vi "Limit Switch Check.vi"(11 "Input Cluster":T1) -> (3 "Output Cluster":T1)   [LabVIEW 2019]
uses:
  Implementation/Turrent Controller Typedef.ctl
  <vilib>/Rock Robotics/WPI/MotorControl/WPI_MotorControlDeviceRef.ctl
  <vilib>/Rock Robotics/WPI/MotorControl/WPI_MotorControlType.ctl
  <vilib>/Rock Robotics/SystemInterfaces/DIO/FPGA_DIOPWMChannel.ctl
  <vilib>/Rock Robotics/WPI/PWM/WPI_PWMDeadband.ctl
  <vilib>/Rock Robotics/SystemInterfaces/DIO/FPGA_DIOChannel.ctl
  <vilib>/Rock Robotics/SystemInterfaces/DutyCycle/FPGA_DutyCycleDevRef.ctl
  <vilib>/Rock Robotics/SystemInterfaces/DutyCycle/FPGA_DutyCycleIndex.ctl
  <vilib>/Rock Robotics/WPI/Counter/WPI_CounterDevRef.ctl
  <vilib>/Rock Robotics/SystemInterfaces/Counter/FPGA_CounterCtrSystemIndex.ctl
  <vilib>/Rock Robotics/WPI/ThirdParty/REV Robotics/SPARK MAX/Typedef/Spark MAX Control Type.ctl
  Support Code/Indicator LED Indexes.ctl
  Support Code/Indicator LED - Green.ctl
panel:
  out "Hard Limit Fwd":bool
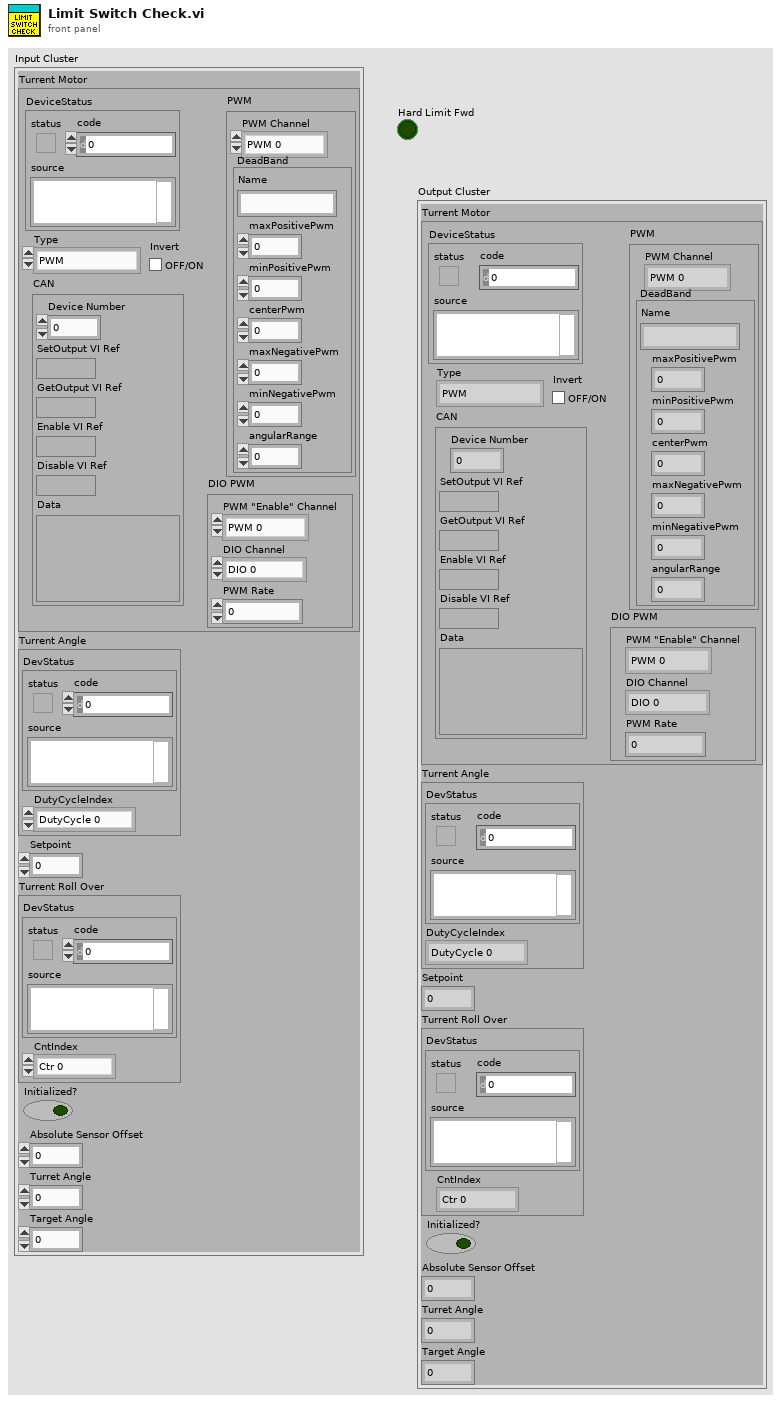
[diagram p1: front panel]
types:
  T1 = typedef "Turrent Controller Typedef.ctl" = cluster{"Turrent Motor":T2, "Turrent Angle":T7, "Setpoint":dbl, "Turrent Roll Over":T9, "Initialized?":bool, "Absolute Sensor Offset":dbl, "Turret Angle":dbl, "Target Angle":dbl}
  T2 = typedef "WPI_MotorControlDeviceRef.ctl" = cluster{"DeviceStatus":errorcluster, "Type":T3, "PWM":cluster{"PWM Channel":T4, "DeadBand":T5}, "CAN":cluster{"Device Number":u8, "SetOutput VI Ref":variant, "GetOutput VI Ref":variant, "Enable VI Ref":variant, "Disable VI Ref":variant, "Data":variant}, "Invert":bool, "DIO PWM":cluster{"PWM \"Enable\" Channel":T4, "DIOChannel":T6, "PWM Rate":dbl}}
  T3 = typedef "WPI_MotorControlType.ctl" = enum16{"PWM", "CAN", "DIO PWM"}
  T4 = typedef "FPGA_DIOPWMChannel.ctl" = enum8{"PWM 0", "PWM 1", "PWM 2", "PWM 3", "PWM 4", "PWM 5", "PWM 6", "PWM 7", "PWM 8", "PWM 9", "PWM MXP 0", "PWM MXP 1", "PWM MXP 2", "PWM MXP 3", "PWM MXP 4", "PWM MXP 5", "PWM MXP 6", "PWM MXP 7", "PWM MXP 8", "PWM MXP 9", "Invalid"}
  T5 = typedef "WPI_PWMDeadband.ctl" = cluster{"Name":string, "maxPositivePwm":i32, "minPositivePwm":i32, "centerPwm":i32, "maxNegativePwm":i32, "minNegativePwm":i32, "angularRange":u16}
  T6 = typedef "FPGA_DIOChannel.ctl" = enum8{"DIO 0", "DIO 1", "DIO 2", "DIO 3", "DIO 4", "DIO 5", "DIO 6", "DIO 7", "DIO 8", "DIO 9", "DIO MXP 0", "DIO MXP 1", "DIO MXP 2", "DIO MXP 3", "DIO MXP 4", "DIO MXP 5", "DIO MXP 6", "DIO MXP 7", "DIO MXP 8", "DIO MXP 9", "DIO MXP 10", "DIO MXP 11", "DIO MXP 12", "DIO MXP 13", "DIO MXP 14", "DIO MXP 15", "SPI Port CS1", "SPI Port CS2", "SPI Port CS3", "SPI Port MISO", "SPI Port MOSI", "Invalid"}
  T7 = typedef "FPGA_DutyCycleDevRef.ctl" = cluster{"DevStatus":errorcluster, "DutyCycleIndex":T8}
  T8 = typedef "FPGA_DutyCycleIndex.ctl" = enum8{"DutyCycle 0", "DutyCycle 1", "DutyCycle 2", "DutyCycle 3", "DutyCycle 4", "DutyCycle 5", "DutyCycle 6", "DutyCycle 7", "Invalid"}
  T9 = typedef "WPI_CounterDevRef.ctl" = cluster{"DevStatus":errorcluster, "CntIndex":T10}
  T10 = typedef "FPGA_CounterCtrSystemIndex.ctl" = enum8{"Ctr 0", "Ctr 1", "Ctr 2", "Ctr 3", "Ctr 4", "Ctr 5", "Ctr 6", "Ctr 7", "Invalid"}
  T11 = typedef "Spark MAX Control Type.ctl" = enum16{"Percent VBus", "Voltage", "Velocity", "Position", "Smart Motion", "Current", "Smart Velocity"}
  T12 = typedef "Indicator LED - Green.ctl" = u32
  T13 = typedef "Indicator LED Indexes.ctl" = enum16{"Code Started", "DS Connected", "Limelight", "Turret Calibrated", "Gyro Calibrated", "USB0 Connected", "USB1 Connected", "FMS Attached"}
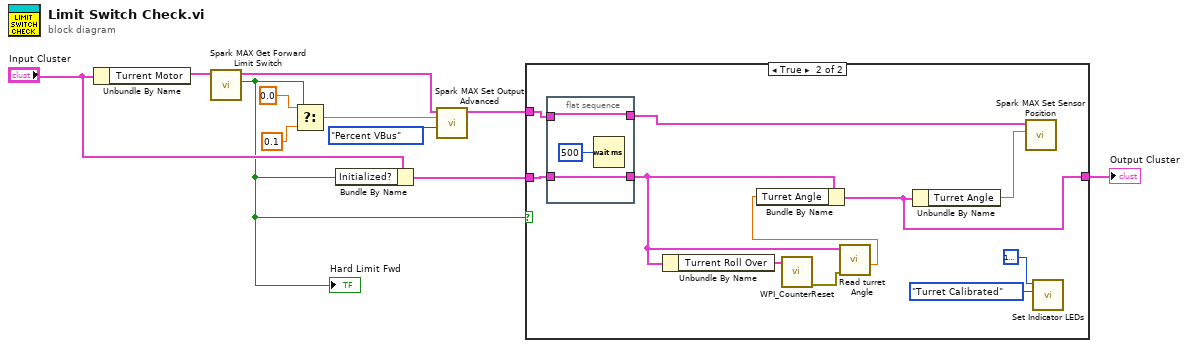
[diagram p0: block diagram]
diagram:
  n1 = Unbundle By Name("Input Cluster") -> ("Turrent Motor"=w7:T2)
  n2 = call <vilib>:"Spark MAX Get Forward Limit Switch.vi"("MotorControlDevRef in"=w7) -> ("Hard Limit Fwd"=w3:bool, "MotorControlDevRef out"=w2:T2)  [unwired: 7 in, 2 out]
  "Hard Limit Fwd" <- w3
  n3 = Select(t=0.0, s=w3, f=0.1) -> (s? t:f=w6:dbl)
  n4 = Bundle By Name(cluster="Input Cluster", "Initialized?"=w3) -> (w5:T1)
  n5 = call <vilib>:"Spark MAX Set Output Advanced.vi"("Control Mode"=Spark_MAX_Control_Type."Percent VBus", "Setpoint"=w6, "MotorControlDevRef"=w2) -> ("MotorControlDevRef"=w1:T2)  [unwired: 7 in, 1 out]
  n6 = case shown="True" w3 {
    tunnel: w5 -> [w12 w22]
    tunnel: [w12 w19] -> w4
    tunnel: w1 -> [_ w23]
    frame False {
    }
    frame True {
      n7 = flat-sequence {
        tunnel: w23 -> [w25]
        tunnel: [w25] -> w21
        tunnel: [w24] -> w16
        tunnel: w22 -> [w24]
        frame #0 {
          n8 = Wait (ms)(milliseconds to wait=u32 500) -> ()  [unwired: 1 out]
        }
      }
      n9 = Unbundle By Name(w16) -> ("Turrent Roll Over"=w18:T9)
      n10 = call <vilib>:"WPI_CounterReset.vi"("CounterDevRef in"=w18) -> ("error out"=w17:errorcluster)  [unwired: 9 in, 1 out]
      n11 = call "Read turret Angle.vi"("error in (no error)"=w17, "Input cluster"=w16) -> ("Turret Angle"=w15:dbl)  [unwired: 6 in, 3 out]
      n12 = Bundle By Name(cluster=w16, "Turret Angle"=w15) -> (w19:T1)
      n13 = Unbundle By Name(w19) -> ("Turret Angle"=w20:dbl)
      n14 = call <vilib>:"Spark MAX Set Sensor Position.vi"("Position"=w20, "MotorControlDeviceRef"=w21) -> ()  [unwired: 8 in, 2 out]
      n15 = call "Set Indicator LEDs.vi"("LED Index"=Indicator_LED_Indexes."Turret Calibrated", "Color"=T12 1851904) -> ()  [unwired: 9 in, 1 out]
    }
  }
  "Output Cluster" <- w4
